vi "Set Count Behaviour.vi"(8 "error in (no error)":errorcluster, 10 "Count Behaviour":T1, 11 "Test Actor API":refnum<class "Test Actor API.lvclass">) -> (0 "error out":errorcluster)   [LabVIEW 2020, in "Test Actor API.lvclass"]
uses:
  Test Actor API.lvclass
  Actor/Count Behaviour.ctl
  C:/Users/neilp/Desktop/Actors/Actor/API/Actor API.lvclass
  Base Actor/API/Actor API.lvclass
  Actor/Test Actor.lvclass
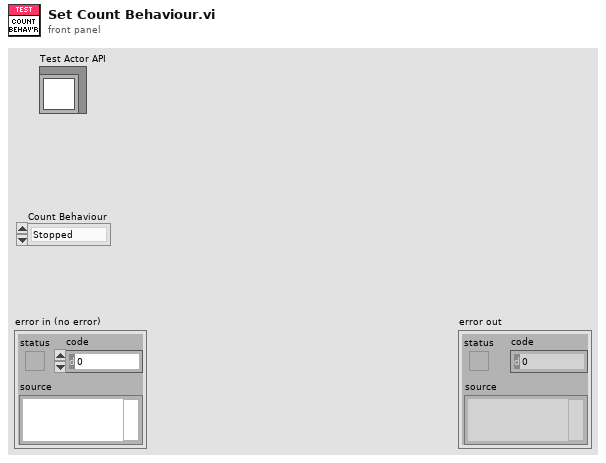
[diagram p1: front panel]
types:
  T1 = typedef "Test Actor.lvclass/Count Behaviour.ctl" = enum16{"Stopped", "Up", "Down"}
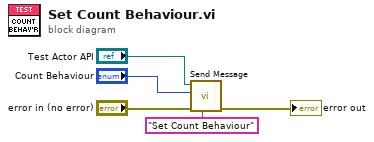
[diagram p0: block diagram]
diagram:
  n1 = call "Send Message.vi"("Name"="Set Count Behaviour", "error in (no error)"="error in (no error)", "Payload"="Count Behaviour", "Actor API in"="Test Actor API") -> ("error out"=→"error out":errorcluster)  [unwired: 7 in]
